vi "Send Virtual Camera Start Stream.vi"(0 "Message Enqueuer":refnum<class "Message Enqueuer.lvclass">, 1 "Message Priority (Normal)":T2=enum."Normal", 5 "Camera Settings":T1={"Exposure Time (ms)"=100.0, "Binning"=enum."2x2", "Scan Mode"=0, "Frames to Acquire"=1000.0, "Pixel Correction"=FALSE, "Frames to Skip"=0, "File Path"=path "", "Duty cycle"=0.0, "ALEX"=FALSE, "Shutter Enable"=[]} {"Exposure Time (ms)" min=1.0 max=10000.0 step=1.0}, 11 "error in (no error)":errorcluster) -> (4 "Message Enqueuer out":refnum<class "Message Enqueuer.lvclass">, 15 "error out":errorcluster)   [LabVIEW 2018, in "Virtual Camera.lvlib" / "Virtual Camera Start Stream Msg.lvclass"]
doc: "This VI sends the message to an actor."
uses:
  Virtual Camera Start Stream Msg.lvclass
  <vilib>/ActorFramework/Message Enqueuer/Message Enqueuer.lvclass
  <vilib>/ActorFramework/Message Enqueuer/Message Priority.ctl
  Resources/Type Defs/Camera Settings.ctl
  C:/Program Files/National Instruments/LabVIEW 2018/vi.lib/ActorFramework/Message/Message.lvclass
  Virtual Camera Start Stream Msg.lvclass/Virtual Camera Start Stream Msg.ctl
  <vilib>/ActorFramework/Message Enqueuer/Message Enqueuer.lvclass/Message Enqueuer.ctl
  <vilib>/ActorFramework/Message Priority Queue/Priority Enqueue.vi
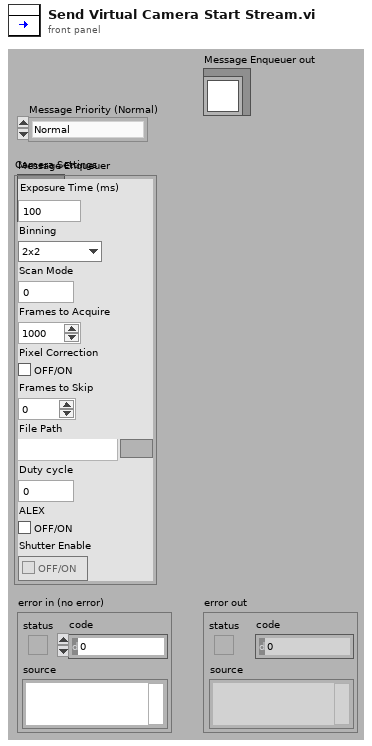
[diagram p1: front panel]
types:
  T1 = typedef "Camera Settings.ctl" = cluster{"Exposure Time (ms)":dbl, "Binning":enum16{"1x1", "2x2", "4x4"}, "Scan Mode":i32, "Frames to Acquire":dbl, "Pixel Correction":bool, "Frames to Skip":u32, "File Path":path, "Duty cycle":dbl, "ALEX":bool, "Shutter Enable":bool[]}
  T2 = typedef "Actor Framework.lvlib/Message Enqueuer.lvclass/Message Priority.ctl" = enum16{"Low", "Normal", "High"}
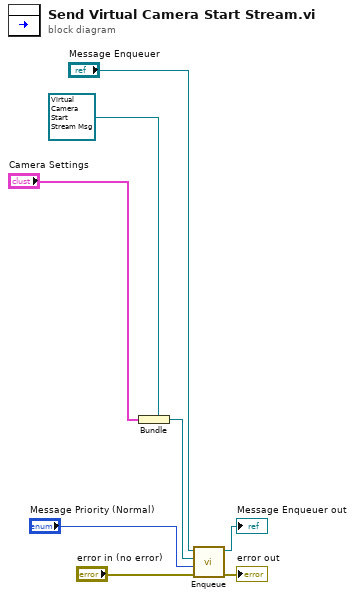
[diagram p0: block diagram]
diagram:
  n1 = Bundle(cluster=refnum<class "Virtual Camera Start Stream Msg.lvclass"> refnum ("Object"), "Camera Settings") -> (w4:refnum<class "Virtual Camera Start Stream Msg.lvclass">)
  n2 = call <vilib>:"Enqueue.vi"("error in (no error)"="error in (no error)", "Message Priority (Normal)"="Message Priority (Normal)", "Message"=w4, "Message Enqueuer in"="Message Enqueuer") -> ("error out"=→"error out":errorcluster, "Message Enqueuer out"=→"Message Enqueuer out":refnum<class "Message Enqueuer.lvclass">)  [unwired: 6 in]
